vi "RSZVB Calibration Standards Catalog.vi"(8 "error in (no error)":errorcluster {"code" format="%.0x"}, 10 "Calibration Kit Name (\"\")":string, 11 "VISA session":refnum<visa-resource-name>) -> (0 "error out":errorcluster {"code" format="%.0x"}, 1 "Catalog":string, 3 "dup VISA session":refnum<visa-resource-name>)   [LabVIEW 2011]
doc: "This VI returns a list of all standards in a given calibration kit.\n\nRemote-control command(s):\n[SENSe<Ch>:]CORRection:CKIT:STANdard:CATalog? '<Ckit_Name>'"
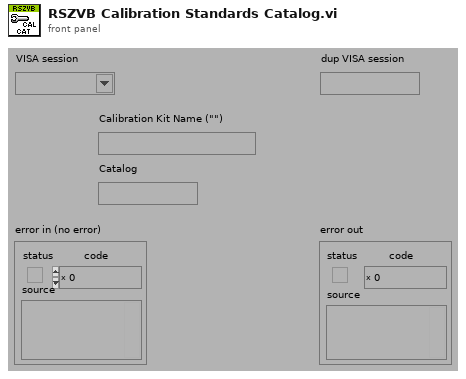
[diagram p1: front panel]
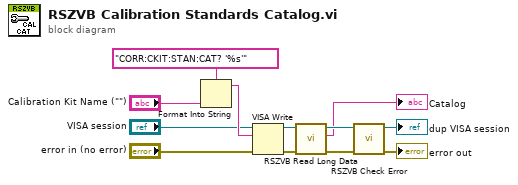
[diagram p0: block diagram]
diagram:
  n1 = Format Into String(format string="CORR:CKIT:STAN:CAT? '%s'", "Calibration Kit Name (\"\")") -> (resulting string=w11:string)  [unwired: 2 in, 1 out]
  n2 = VISA Write(VISA resource name="VISA session", write buffer=w11, error in (no error)="error in (no error)") -> (VISA resource name out=w2:refnum<visa-resource-name>, error out=w3:errorcluster)  [unwired: 1 out]
  n3 = call "RSZVB Read Long Data.vi"("error in (no error)"=w3, "VISA resource name"=w2) -> ("error out"=w4:errorcluster, "Data"=→"Catalog":string, "VISA resource name out"=w5:refnum<visa-resource-name>)  [unwired: 7 in]
  n4 = call "RSZVB Check Error.vi"("error in (no error)"=w4, "VISA session"=w5) -> ("error out"=→"error out":errorcluster, "dup VISA session"=→"dup VISA session":refnum<visa-resource-name>)  [unwired: 8 in]
